vi "Exp no 5a Binary to Gray Conversion.vi"() -> ()   [LabVIEW 2010]
panel:
  in  "B4":bool
  in  "B3":bool
  out "G4":bool
  out "G3":bool
  out "G2":bool
  out "G1":bool
  in  "B2":bool
  in  "B1":bool
  # "BINARY CODE TO GRAY CODE CONVERSION"
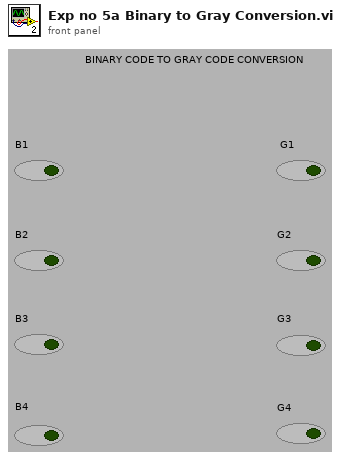
[diagram p1: front panel]
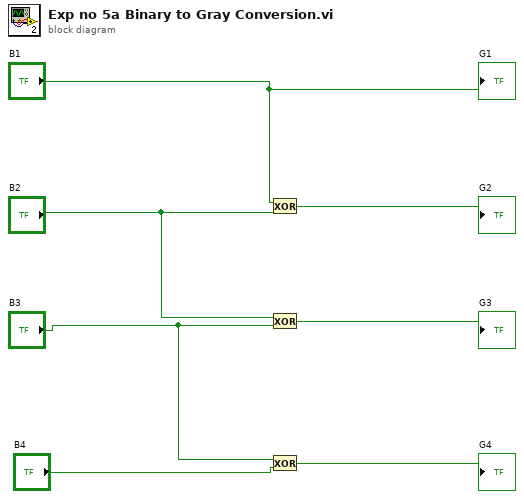
[diagram p0: block diagram]
diagram:
  n1 = Exclusive Or(1:"B2", 2:"B1") -> (0:→"G2":bool)
  n2 = Exclusive Or(1:"B3", 2:"B2") -> (0:→"G3":bool)
  n3 = Exclusive Or(1:"B4", 2:"B3") -> (0:→"G4":bool)
  "G1" <- "B1"
